vi "AINetworkInterface.vi"(0 "Server Port":u16=12500, 1 "Server Address":string="127.0.0.1") -> ()   [LabVIEW 2025]
uses:
  <vilib>/net/WFCN/NI_WFCN.lvlib
panel:
  out "error out":errorcluster
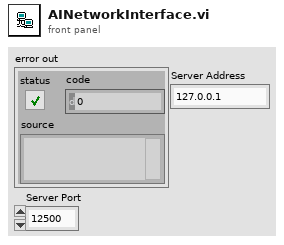
[diagram p1: front panel]
types:
  T1 = typedef "NI_WFCN.lvlib/Network Status.ctl" = enum16{"Indeterminate", "Configured", "Unconfigured"}
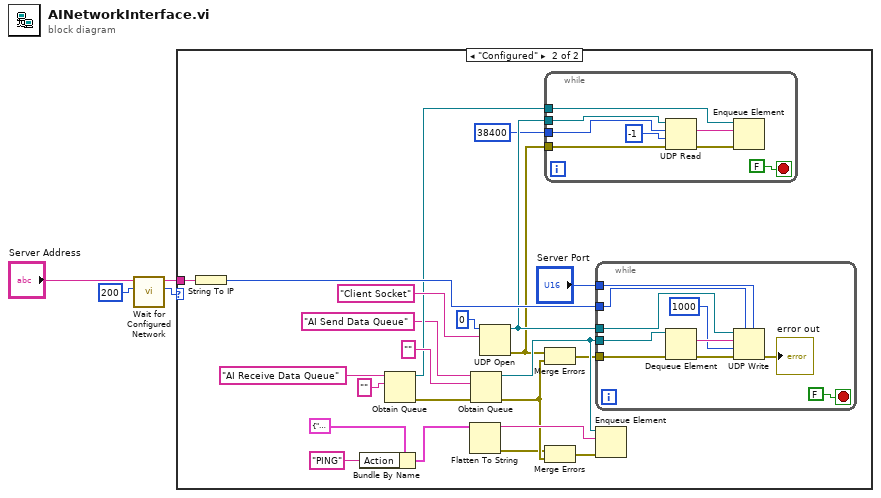
[diagram p0: block diagram]
diagram:
  n1 = call <vilib>:"Wait for Configured Network.vi"("timeout in ms"=200, "hostname or URL in"="Server Address") -> ("network status for remote host"=w1:T1, "hostname or URL out"=w3:string)  [unwired: 8 in]
  n2 = case shown="\"Configured\"" w1 {
    tunnel: w3 -> [_ w23]
    frame "Indeterminate", Default {
    }
    frame "Configured" {
      n3 = String To IP(1:w23) -> (0:w24:u32)
      n4 = Bundle By Name(cluster=cluster{"Action":string, "Data":string} {"Action"="", "Data"=""} ("CommandCluster"), "Action"="PING" ("element")) -> (w12:cluster{"Action":string, "Data":string})
      n5 = Obtain Queue(name (unnamed)="AI Receive Data Queue", element data type="") -> (queue out=w16:refnum<queue>, error out=w18:errorcluster)  [unwired: 3 in, 1 out]
      n6 = Flatten To String(anything=w12) -> (data string=w11:string, error out=w7:errorcluster)  [unwired: 3 in, 1 out]
      n7 = Obtain Queue(name (unnamed)="AI Send Data Queue", element data type="" ("Data"), error in (no error)=w18) -> (queue out=w17:refnum<queue>, error out=w9:errorcluster)  [unwired: 2 in, 1 out]
      n8 = UDP Open(10:"Client Socket" ("service name"), 11:u16 0 ("port")) -> (port=w20:refnum<k16>, 0:w15:errorcluster)  [unwired: 3 in, 1 out]
      n9 = while {
        tunnel: w16 -> [w45]
        tunnel: w20 -> [w41]
        tunnel: 38400 ("max size (548)") -> [w40]
        tunnel: w15 -> [w38]
        stop <- FALSE stop-if-true
        n10 = UDP Read(connection ID=w41, max size (548)=w40, timeout ms (25000)=-1, 8:w38) -> (data out=w44:string, error out=w39:errorcluster)  [unwired: 3 out]
        n11 = Enqueue Element(queue=w45, element=w44, error in (no error)=w39) -> ()  [unwired: 1 in, 3 out]
      }
      n12 = Merge Errors(w15, w9) -> (w10:errorcluster)
      n13 = Merge Errors(w7, w9) -> (w8:errorcluster)
      n14 = while {
        tunnel: w17 -> [w37]
        tunnel: w24 -> [w34]
        tunnel: "Server Port" -> [w33]
        tunnel: w20 -> [w30]
        tunnel: w10 -> [w29]
        stop <- FALSE stop-if-true
        n15 = Dequeue Element(queue=w37, error in (no error)=w29) -> (element=w36:string, error out=w28:errorcluster)  [unwired: 1 in, 2 out]
        n16 = UDP Write(address=w34, port or service name=w33, connection ID=w30, data in=w36, 8:w28, 9:1000 ("timeout ms (25000)")) -> (error out=→"error out":errorcluster)  [unwired: 1 out]
      }
      n17 = Enqueue Element(queue=w17, element=w11, error in (no error)=w8) -> ()  [unwired: 1 in, 3 out]
    }
  }
